vi "ParseShortcut.vi"(8 "error in (no error)":errorcluster, 11 "text in":refnum<class "text.lvclass">) -> (0 "error out":errorcluster, 3 "text out":refnum<class "text.lvclass">)   [LabVIEW 2009, in "text.lvclass"]
uses:
  text.lvclass
  text.lvclass/text.ctl
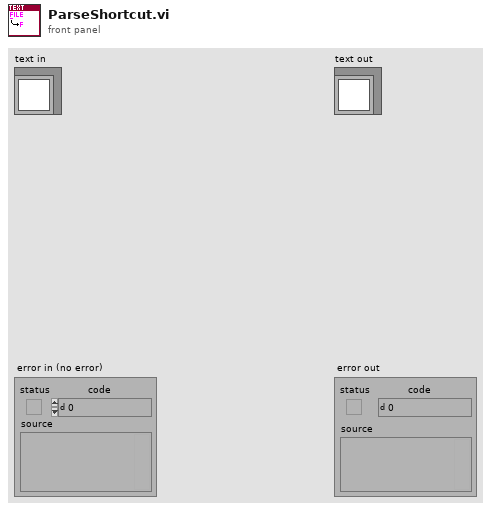
[diagram p1: front panel]
types:
  T1 = enum16{"Type?", "Plain", "Underline", "Parentheses", "End"}
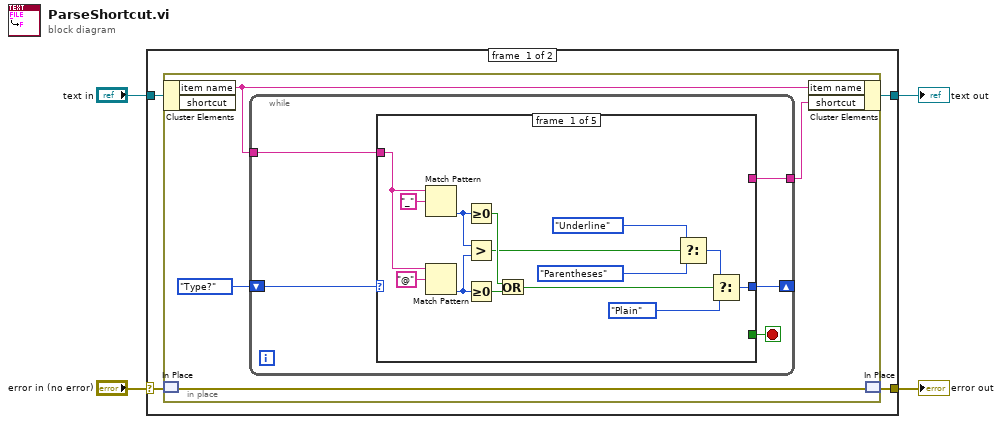
[diagram p0: block diagram]
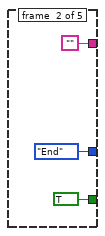
[diagram p2: hidden frame]
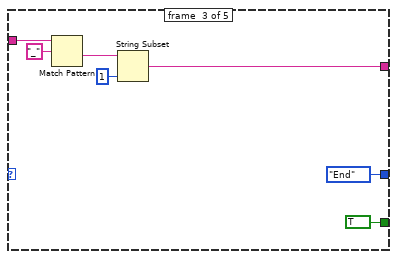
[diagram p3: hidden frame]
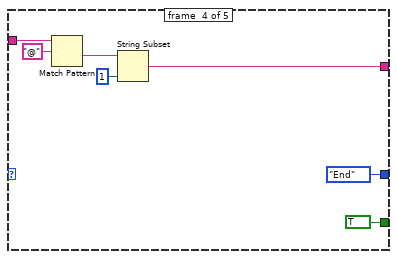
[diagram p4: hidden frame]
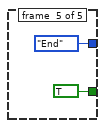
[diagram p5: hidden frame]
diagram:
  n1 = case shown="No Error" "error in (no error)" {
    selector: "error in (no error)" -> [w6 w52]
    tunnel: [w5 w52] -> w1
    tunnel: [w8 w51] -> w3
    tunnel: "text in" -> [w7 w51]
    frame #0 {
      n2 = in-place {
        n3 = in-place-cluster #1(w7) -> ("item name"=w11:string)  [unwired: 1 out]
        n4 = in-place-match #2(w6) -> (w10:errorcluster)
        n5 = while {
          shift-right: [w16] -> _
          shift-left: T1."Type?" ("state") -> [w17]
          tunnel: w11 -> [w15]
          tunnel: [w13] -> w9
          stop <- w14 stop-if-true
          n6 = case shown="\"Underline\"" w17 {
            tunnel: [w30 T1."End" ("state") T1."End" ("state") T1."End" ("state") T1."End" ("state")] -> w16
            tunnel: w15 -> [w26 _ w38 w45 _]
            tunnel: [_ TRUE TRUE TRUE TRUE] -> w14
            tunnel: [_ "" w35 w42 _] -> w13
            frame #0 {
              n7 = Match Pattern(string=w26, regular expression="_") -> (offset past match=w19:i32)  [unwired: 1 in, 3 out]
              n8 = Match Pattern(string=w26, regular expression="@") -> (offset past match=w18:i32)  [unwired: 1 in, 3 out]
              n9 = Greater Or Equal To 0?(x=w19) -> (x >= 0?=w23:bool)
              n10 = Greater?(x=w19, y=w18) -> (0:w20:bool)
              n11 = Greater Or Equal To 0?(x=w18) -> (x >= 0?=w24:bool)
              n12 = Or(x=w23, y=w24) -> (x .or. y?=w25:bool)
              n13 = Select(t=T1."Underline" ("state"), s=w20, f=T1."Parentheses" ("state")) -> (s? t:f=w27:T1)
              n14 = Select(t=w27, s=w25, f=T1."Plain" ("state")) -> (s? t:f=w30:T1)
            }
            frame #1 {
            }
            frame #2 {
              n15 = Match Pattern(string=w38, regular expression="_") -> (after substring=w39:string)  [unwired: 1 in, 3 out]
              n16 = String Subset(string=w39, length (rest)=1 ("length (rest)")) -> (substring=w35:string)  [unwired: 1 in]
            }
            frame #3 {
              n17 = Match Pattern(string=w45, regular expression="@") -> (after substring=w46:string)  [unwired: 1 in, 3 out]
              n18 = String Subset(string=w46, length (rest)=1 ("length (rest)")) -> (substring=w42:string)  [unwired: 1 in]
            }
            frame #4 {
            }
          }
        }
        n19 = in-place-cluster #1("item name"=w11, "shortcut"=w9) -> (w8:refnum<class "text.lvclass">)
        n20 = in-place-match #2(w10) -> (w5:errorcluster)
      }
    }
    frame #1 {
    }
  }
  "text out" <- w3
  "error out" <- w1
